vi "Add Control to Cluster (from src ref) Ret Created Control.vi"(7 "New Control Label":string, 8 "error in (no error)":errorcluster, 9 "Cluster ref in (owner)":refnum<vi>, 10 "Source control ref in":refnum<vi>, 11 "Owning VI ref in":refnum<vi>) -> (0 "error out":errorcluster, 1 "Cluster ref out (owner)":refnum<vi>, 2 "Control ref out":refnum<vi>, 3 "Owning VI ref out":refnum<vi>)   [LabVIEW 2019, in "gRPC Template Creation Utility.lvlib"]
uses:
  gRPC Template Creation Utility.lvlib
  <vilib>/Utility/miscctls.llb/LVPositionTypeDef.ctl
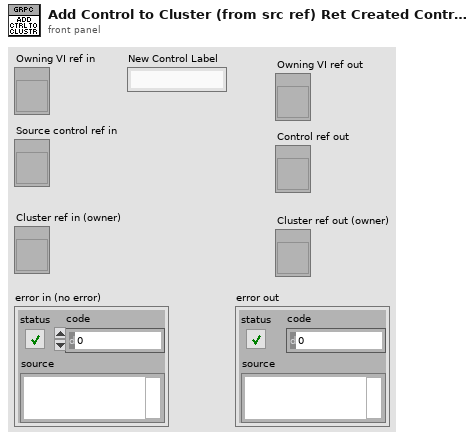
[diagram p1: front panel]
types:
  T1 = typedef "LVPositionTypeDef.ctl" = cluster{"Left":i32, "Top":i32}
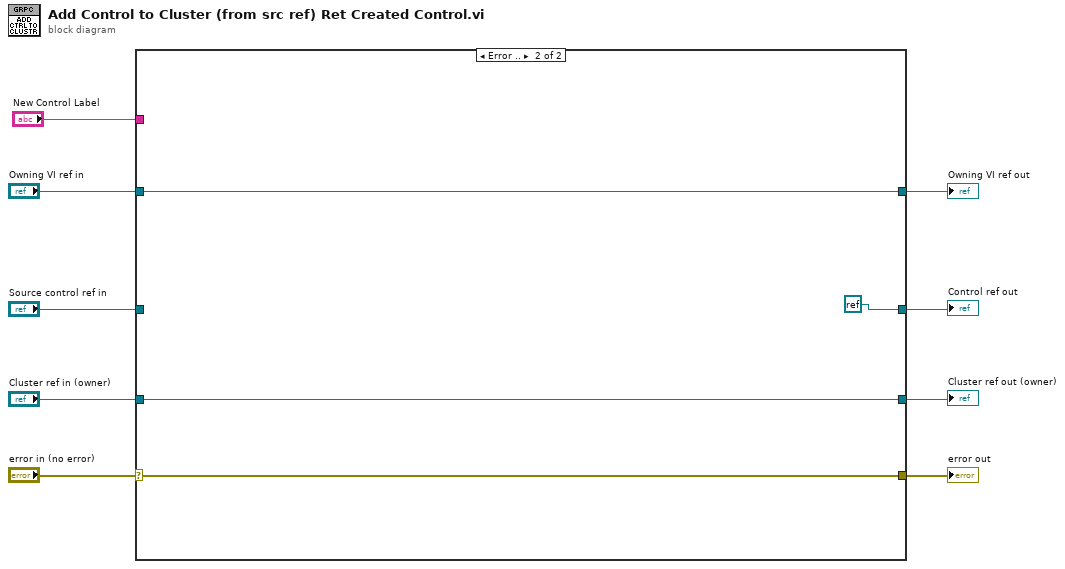
[diagram p0: block diagram]
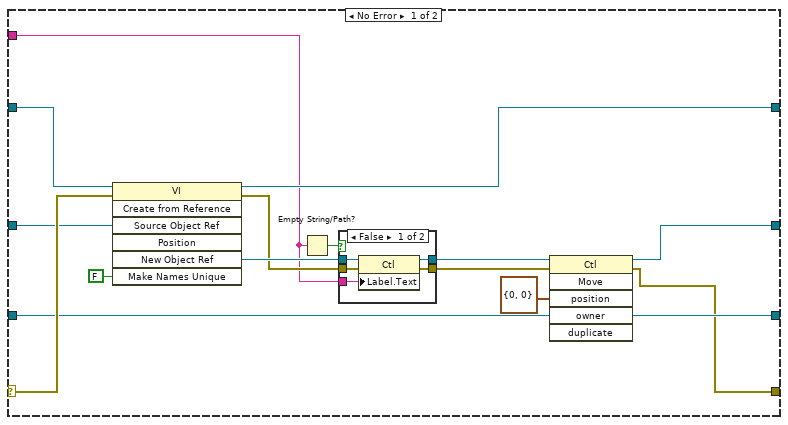
[diagram p2: hidden frame]
diagram:
  n1 = case shown="Error .." "error in (no error)" {
    selector: "error in (no error)" -> [w20 w33]
    tunnel: [w24 w35] -> w9
    tunnel: "Owning VI ref in" -> [w23 w35]
    tunnel: "Source control ref in" -> [w19 _]
    tunnel: "Cluster ref in (owner)" -> [w18 w34]
    tunnel: [w11 w33] -> w5
    tunnel: [w10 refnum<k0> refnum] -> w3
    tunnel: [w18 w34] -> w2
    tunnel: "New Control Label" -> [w13 _]
    frame No Error {
      n2 = invoke class="VI" method="Create from Reference"(reference=w23, error in=w20, "Source Object Ref"=w19, "Make Names Unique"=FALSE ("Make Names Unique (F)")) -> (reference out=w24:refnum<vi>, error out=w15:errorcluster, "New Object Ref"=w17:refnum<vi>)  [unwired: 3 in, 4 out]
      n3 = Empty String/Path?(string/path=w13) -> (empty?=w12:bool)
      n4 = case shown="False" w12 {
        tunnel: w17 -> [w29 w31]
        tunnel: [w28 w31] -> w16
        tunnel: w13 -> [w27 _]
        tunnel: w15 -> [w26 w30]
        tunnel: [w25 w30] -> w14
        frame False {
          n5 = property class="Ctl"(reference=w29, error in=w26, "Label.Text"=w27) -> (reference out=w28:refnum<vi>, error out=w25:errorcluster)
        }
        frame True {
        }
      }
      n6 = invoke class="Ctl" method="Move"(reference=w16, error in=w14, "position"=T1 {"Left"=0, "Top"=0}, "owner"=w18) -> (reference out=w10:refnum<vi>, error out=w11:errorcluster)  [unwired: 2 in, 4 out]
    }
    frame Error {
    }
  }
  "error out" <- w5
  "Owning VI ref out" <- w9
  "Control ref out" <- w3
  "Cluster ref out (owner)" <- w2
